vi "PPMS_CREA_SECUENCIA_REPITE.vi"(8 "error in (no error)":errorcluster) -> (0 "error out":errorcluster, 1 "Total":string[](array[string]), 2 "Pasos":i32, 3 "Secuencia":string[](array[string]), 4 "Secuciclos":string[](array[string]), 6 "Pasos f":i32)   [LabVIEW 2017]
uses:
  <vilib>/Utility/file.llb/Read Delimited Spreadsheet (string).vi
panel:
  out "idxScanVi":i16
  out "idxScanVf":i16
  out "Scan V":bool
  out "subArray2D":string[][](array[string])
  out "Seq scans":string[](array[string])
  out "Seq final":string[](array[string])
  out "Seq inicial":string[](array[string])
  out "idxScanTi":i16
  out "idxScanFi":i16
  out "idxScanFf":i16
  out "idxScanTf":i16
  out "Array2D":string[][](array[string])
  out "Scan T":bool
  out "Scan F":bool
  in  "Salir":bool
  in  "Borra linea":bool
  in  "Grabar":bool
  in  "Cargar":bool
  out "SequenceFile":path
  in  "Command line (double click)":i32(listbox) caption="Válvulas"
  in  "Secuencia":i32(listbox)=-1
  # "Noviembre 2020 V1.4  a-sslcdms"
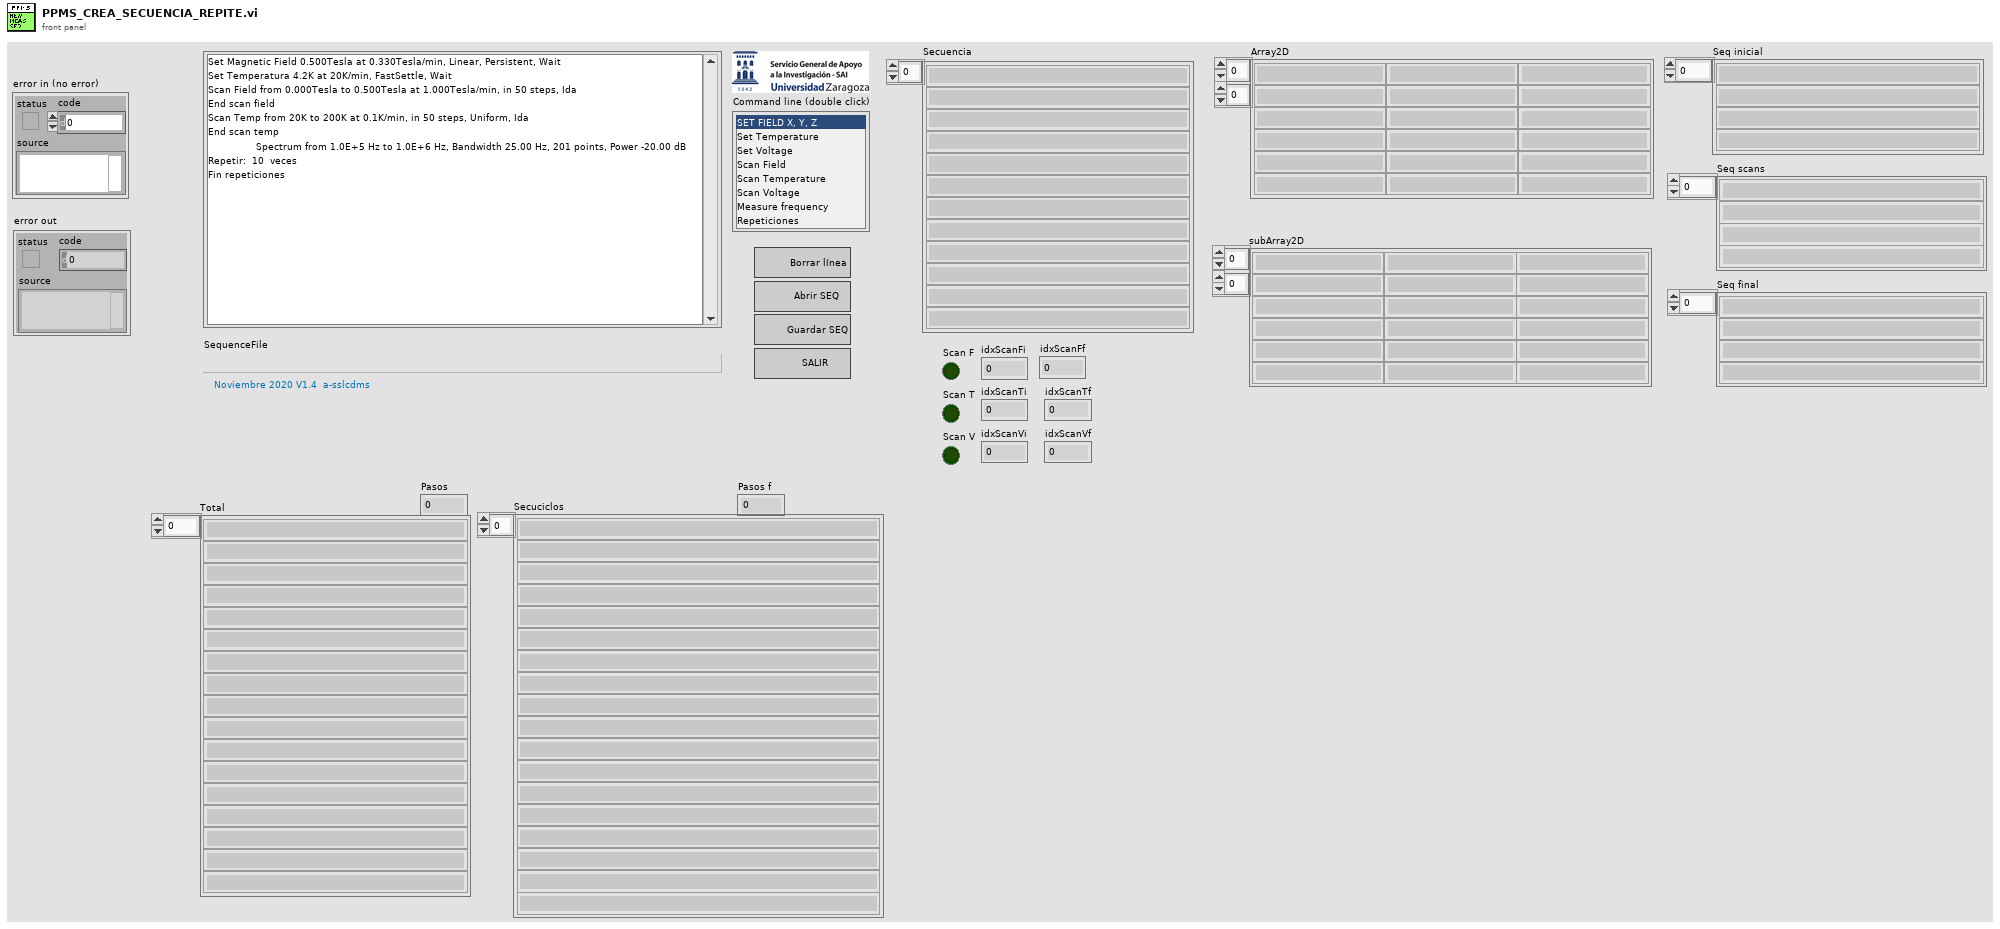
[diagram p1: front panel]
types:
  T1 = enum16{"open", "open or create", "create or replace", "create", "open (read only)"}
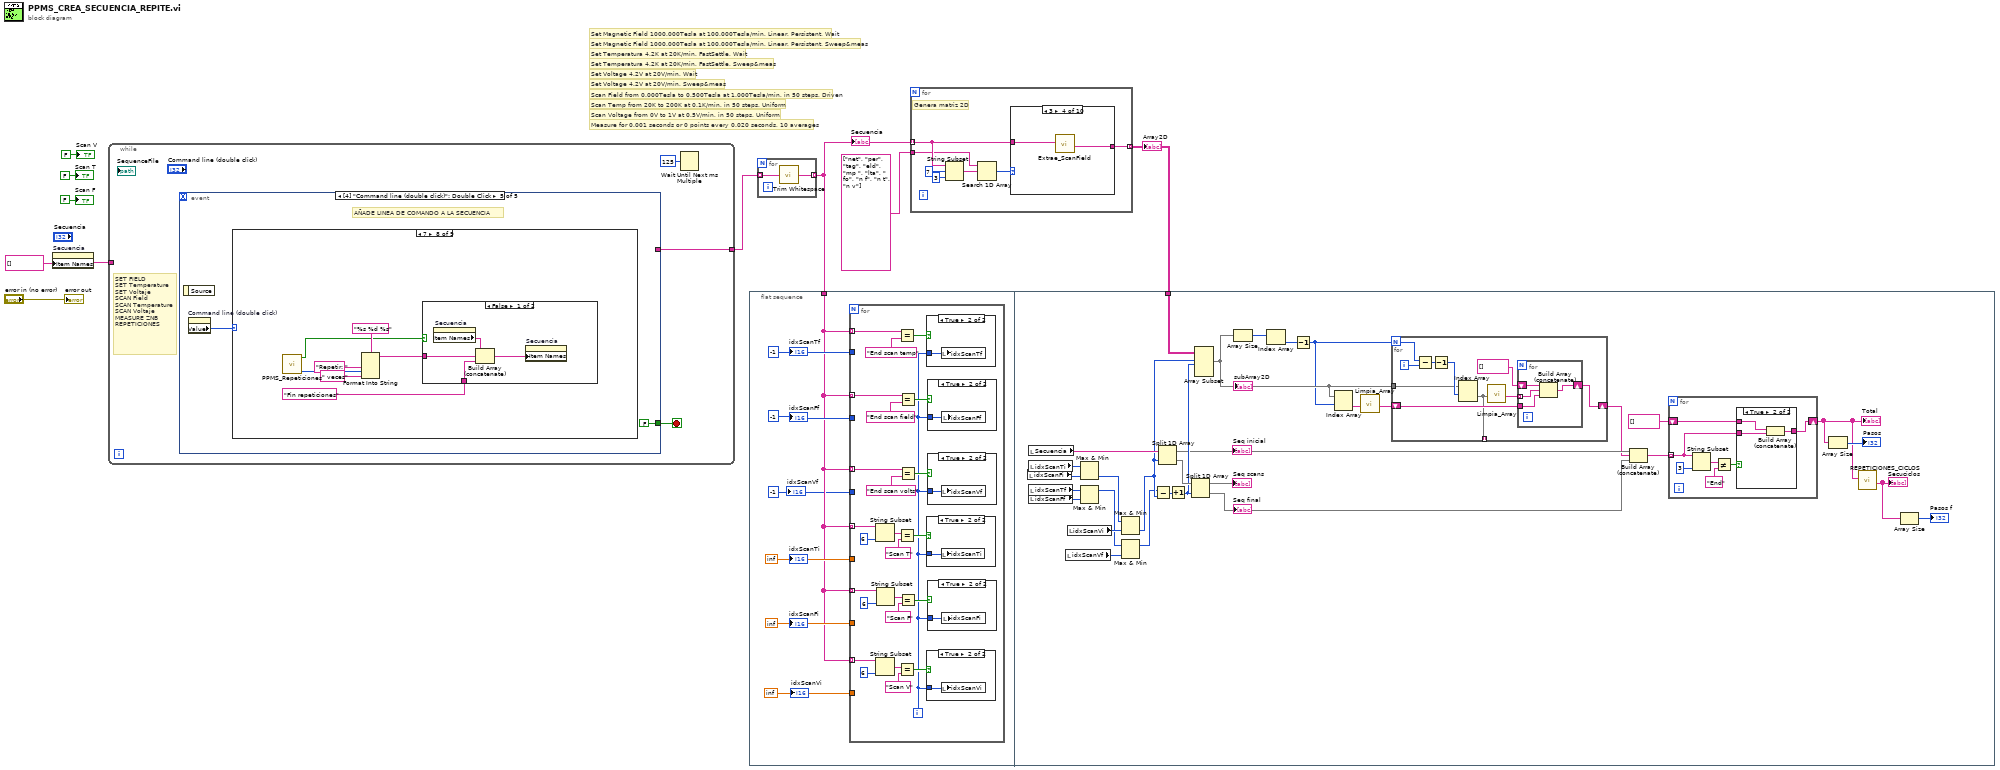
[diagram p0: block diagram]
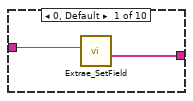
[diagram p9: hidden frame]
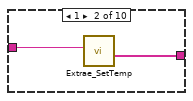
[diagram p10: hidden frame]
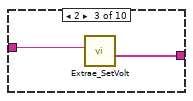
[diagram p11: hidden frame]
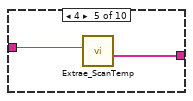
[diagram p12: hidden frame]
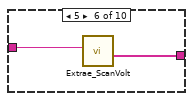
[diagram p13: hidden frame]
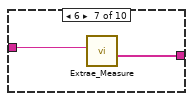
[diagram p14: hidden frame]
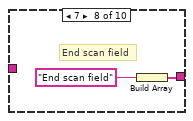
[diagram p15: hidden frame]
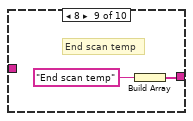
[diagram p16: hidden frame]
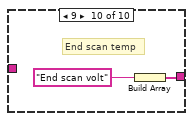
[diagram p17: hidden frame]
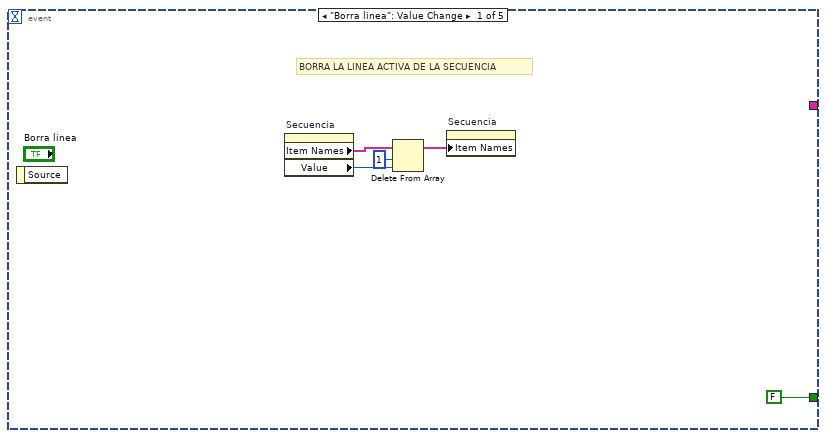
[diagram p18: hidden frame]
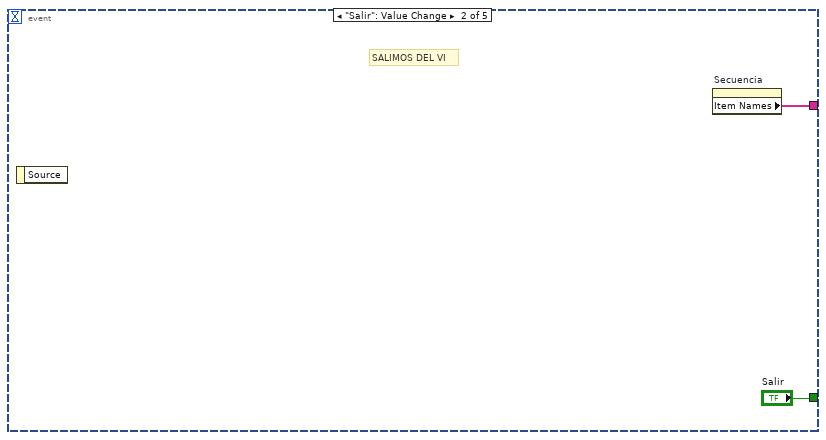
[diagram p19: hidden frame]
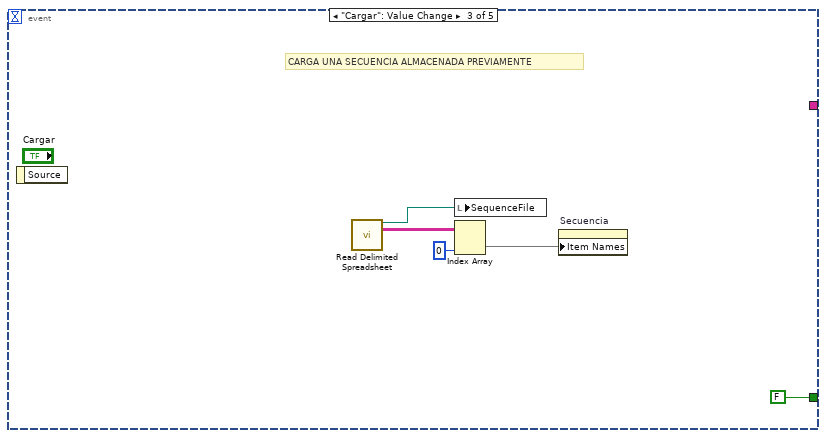
[diagram p20: hidden frame]
diagram:
  w9 = string[] [] ("Item Names")
  # "Measure for 0.001 seconds or 0 points every 0.020 seconds, 10 averages"
  # "Scan Voltage from 0V to 1V at 0.5V/min, in 50 steps, Uniform"
  # "Scan Temp from 20K to 200K at 0.1K/min, in 50 steps, Uniform"
  # "Scan Field from 0.000Tesla to 0.500Tesla at 1.000Tesla/min, in 50 steps, Driven"
  # "Set Temperatura 4.2K at 20K/min, FastSettle, Sweep&meas"
  # "Set Temperatura 4.2K at 20K/min, FastSettle, Wait"
  # "Set Magnetic Field 1000.000Tesla at 100.000Tesla/min, Linear, Persistent, Sweep&meas"
  # "Set Magnetic Field 1000.000Tesla at 100.000Tesla/min, Linear, Persistent, Wait"
  # "Set Voltage 4.2V at 20V/min, Sweep&meas"
  # "Set Voltage 4.2V at 20V/min, Wait"
  n1 = property on="Secuencia" class="LstBox (strict)"("Item Names"=w9) -> ()  [unwired: 2 in, 2 out]
  n2 = while {
    tunnel: w9 -> [_]
    tunnel: [w10] -> w4
    stop <- w11 stop-if-true
    # "SET FIELD\nSET Temperature\nSET Voltaje\nSCAN Field\nSCAN Temperature\nSCAN Voltaje\nMEASURE ZNB\nREPETICIONES"
    n3 = event shown="[4] \"Command line (double click)\": Double Click" {
      selector: _ -> [_ _ _ _ _]
      dyn-events: _ -> [_ _ _ _ _]
      timeout: _ -> [_ _ _ _ _]
      tunnel: [FALSE ("Salir") "Salir" FALSE ("Salir") FALSE ("Salir") FALSE ("Salir")] -> w11
      tunnel: [_ w18 _ _ _] -> w10
      event "Borra linea": Value Change {
        # "BORRA LA LINEA ACTIVA DE LA SECUENCIA"
        n4 = event-data() -> ()  [unwired: 1 in, 1 out]
        n5 = property on="Secuencia" class="LstBox (strict)"() -> ("Item Names"=w17:string[], "Value"=w16:i32)  [unwired: 2 in, 2 out]
        n6 = Delete From Array(array=w17, length=1, index=w16) -> (array with subset deleted=w14:string[])  [unwired: 1 out]
        n7 = property on="Secuencia" class="LstBox (strict)"("Item Names"=w14) -> ()  [unwired: 2 in, 2 out]
      }
      event "Salir": Value Change {
        # "SALIMOS DEL VI"
        n8 = event-data() -> ()  [unwired: 1 in, 1 out]
        n9 = property on="Secuencia" class="LstBox (strict)"() -> ("Item Names"=w18:string[])  [unwired: 2 in, 2 out]
      }
      event "Cargar": Value Change {
        # "CARGA UNA SECUENCIA ALMACENADA PREVIAMENTE"
        n10 = event-data() -> ()  [unwired: 1 in, 1 out]
        n11 = call-poly <vilib>:"Read Delimited Spreadsheet.vi"() -> ("new file path (Not A Path if cancelled)"=w21:path, "all rows"=w20:string[][])  [unwired: 10 in, 4 out]
        n12 = local write "SequenceFile"(w21) -> ()
        n13 = Index Array(array=w20, index (col)=0 ("disabled index (col)")) -> (element=w22:string[])  [unwired: 1 in]
        n14 = property on="Secuencia" class="LstBox (strict)"("Item Names"=w22) -> ()  [unwired: 2 in, 2 out]
      }
      event "Grabar": Value Change {
        # "GRABA UNA SECUENCIA PARA USAR MAS ADELANTE"
        n15 = event-data() -> ()  [unwired: 1 in, 1 out]
        n16 = property on="Secuencia" class="LstBox (strict)"() -> ("Item Names"=w28:string[])  [unwired: 2 in, 2 out]
        n17 = call <vilib>:"Open_Create_Replace File.vi"("function (open:0)"=T1."create or replace") -> ("new file path"=w25:path)  [unwired: 7 in, 3 out]
        n18 = local write "SequenceFile"(w25) -> ()
        n19 = for {
          tunnel: w28 -> [w31] mode=indexing
          shift-right: [w33] -> _
          shift-left: w25 -> [w34]
          n20 = Concatenate Strings(w31, "\r\n") -> (w30:string)
          n21 = call <vilib>:"Write Characters To File.vi"("append to file? (new file:F)"=TRUE, "character string"=w30, "file path (dialog if empty)"=w34) -> ("new file path (Not A Path if cancelled)"=w33:path)  [unwired: 2 in]
        }
      }
      event "Command line (double click)": Double Click {
        # "AÑADE LINEA DE COMANDO A LA SECUENCIA"
        n22 = event-data() -> ()  [unwired: 1 in, 1 out]
        n23 = property on="Command line (double click)" class="LstBox (strict)"() -> ("Value"=w35:i32)  [unwired: 2 in, 2 out]
        n24 = case shown="7" w35 {
          frame 0, Default {
            # "SET FIELD"
            n25 = call "PPMS_SetCampo.vi"("Index"=i8 0) -> ("resulting string 1"=w38:string, "Cancelled?"=w39:bool)  [unwired: 6 in, 1 out]
            n26 = case shown="False" w39 {
              tunnel: w38 -> [w40 _]
              frame False {
                n27 = property on="Secuencia" class="LstBox (strict)"() -> ("Item Names"=w41:string[])  [unwired: 2 in, 2 out]
                n28 = Build Array (concatenate)(w41, w40) -> (w42:string[])
                n29 = property on="Secuencia" class="LstBox (strict)"("Item Names"=w42) -> ()  [unwired: 2 in, 2 out]
              }
              frame True {
              }
            }
          }
          frame 1 {
            # "SET TEMPERATURE"
            n30 = call "PPMS_SetTemperatura.vi"("Index"=i8 0) -> ("resulting string 1"=w44:string, "Cancelled?"=w45:bool)  [unwired: 6 in, 1 out]
            n31 = case shown="False" w45 {
              tunnel: w44 -> [w46 _]
              frame False {
                n32 = property on="Secuencia" class="LstBox (strict)"() -> ("Item Names"=w48:string[])  [unwired: 2 in, 2 out]
                n33 = Build Array (concatenate)(w48, w46) -> (w47:string[])
                n34 = property on="Secuencia" class="LstBox (strict)"("Item Names"=w47) -> ()  [unwired: 2 in, 2 out]
              }
              frame True {
              }
            }
          }
          frame 2 {
            # "SET VOLTAGE"
            n35 = case shown="False" FALSE {
              frame False {
                n36 = One Button Dialog(message="Comando desactivado") -> ()  [unwired: 1 in, 1 out]
              }
              frame True {
                n37 = call "PPMS_SetVoltage.vi"("Index"=i8 0) -> ("resulting string 1"=w51:string, "Cancelled?"=w52:bool)  [unwired: 6 in, 1 out]
                n38 = case shown="False" w52 {
                  tunnel: w51 -> [w56 _]
                  frame False {
                    n39 = property on="Secuencia" class="LstBox (strict)"() -> ("Item Names"=w55:string[])  [unwired: 2 in, 2 out]
                    n40 = Build Array (concatenate)(w55, w56) -> (w54:string[])
                    n41 = property on="Secuencia" class="LstBox (strict)"("Item Names"=w54) -> ()  [unwired: 2 in, 2 out]
                  }
                  frame True {
                  }
                }
              }
            }
          }
          frame 3 {
            # "SCAN FIELD"
            n42 = local read "Scan F"() -> (w57:bool)
            n43 = case shown="False" w57 {
              frame False {
                n44 = local read "Scan T"() -> (w63:bool)
                n45 = local read "Scan V"() -> (w64:bool)
                n46 = Select(t=i8 2 ("Index"), s=w63, f=i8 0 ("Index")) -> (s? t:f=w59:i8)
                n47 = Select(t=i8 2 ("Index"), s=w64, f=i8 0 ("Index")) -> (s? t:f=w60:i8)
                n48 = Add(x=w60, y=w59) -> ()  [unwired: 1 out]
                n49 = local write "Scan F"(TRUE ("Scan T")) -> ()
                n50 = call "PPMS_ScanCampo.vi"("Index"=i8 0) -> ("resulting string 2"=w69:string, "resulting string 1"=w70:string, "Cancelled?"=w68:bool)  [unwired: 5 in, 1 out]
                n51 = case shown="False" w68 {
                  tunnel: w70 -> [w75 _]
                  tunnel: w69 -> [w74 _]
                  frame False {
                    n52 = property on="Secuencia" class="LstBox (strict)"() -> ("Item Names"=w73:string[])  [unwired: 2 in, 2 out]
                    n53 = Build Array(w75, w74) -> (w72:string[])
                    n54 = Build Array (concatenate)(w73, w72) -> (w71:string[])
                    n55 = property on="Secuencia" class="LstBox (strict)"("Item Names"=w71) -> ()  [unwired: 2 in, 2 out]
                  }
                  frame True {
                  }
                }
              }
              frame True {
                n56 = One Button Dialog(message="Solo esta permitido\nun scan de campo por secuencia") -> ()  [unwired: 1 in, 1 out]
              }
            }
          }
          frame 4 {
            # "SCAN TEMPERATURE"
            n57 = local read "Scan T"() -> (w77:bool)
            n58 = case shown="False" w77 {
              frame False {
                n59 = local read "Scan V"() -> (w83:bool)
                n60 = local read "Scan F"() -> (w84:bool)
                n61 = local write "Scan T"(TRUE ("Scan T")) -> ()
                n62 = Select(t=i8 2 ("Index"), s=w83, f=i8 0 ("Index")) -> (s? t:f=w79:i8)
                n63 = Select(t=i8 2 ("Index"), s=w84, f=i8 0 ("Index")) -> (s? t:f=w80:i8)
                n64 = Add(x=w80, y=w79) -> ()  [unwired: 1 out]
                n65 = call "PPMS_ScanTemperatura.vi"("Index"=i8 0) -> ("resulting string 2"=w88:string, "resulting string 1"=w89:string, "Cancelled?"=w90:bool)  [unwired: 5 in, 1 out]
                n66 = case shown="False" w90 {
                  tunnel: w89 -> [w95 _]
                  tunnel: w88 -> [w94 _]
                  frame False {
                    n67 = property on="Secuencia" class="LstBox (strict)"() -> ("Item Names"=w93:string[])  [unwired: 2 in, 2 out]
                    n68 = Build Array(w95, w94) -> (w92:string[])
                    n69 = Build Array (concatenate)(w93, w92) -> (w91:string[])
                    n70 = property on="Secuencia" class="LstBox (strict)"("Item Names"=w91) -> ()  [unwired: 2 in, 2 out]
                  }
                  frame True {
                  }
                }
              }
              frame True {
                n71 = One Button Dialog(message="Solo esta permitido\nun scan de temperatura por secuencia") -> ()  [unwired: 1 in, 1 out]
              }
            }
          }
          frame 5 {
            n72 = case shown="True" FALSE {
              frame False {
                n73 = One Button Dialog(message="Comando desactivado") -> ()  [unwired: 1 in, 1 out]
              }
              frame True {
                # "SCAN VOLTAGE"
                n74 = local read "Scan V"() -> (w99:bool)
                n75 = case shown="False" w99 {
                  frame False {
                    n76 = local read "Scan T"() -> (w107:bool)
                    n77 = local read "Scan F"() -> (w108:bool)
                    n78 = local write "Scan V"(TRUE ("Scan T")) -> ()
                    n79 = Select(t=i8 2 ("Index"), s=w107, f=i8 0 ("Index")) -> (s? t:f=w105:i8)
                    n80 = Select(t=i8 2 ("Index"), s=w108, f=i8 0 ("Index")) -> (s? t:f=w106:i8)
                    n81 = Add(x=w106, y=w105) -> ()  [unwired: 1 out]
                    n82 = call "PPMS_ScanVoltage.vi"("Index"=i8 0) -> ("resulting string 2"=w110:string, "resulting string 1"=w111:string, "Cancelled?"=w112:bool)  [unwired: 5 in, 1 out]
                    n83 = case shown="False" w112 {
                      tunnel: w111 -> [w117 _]
                      tunnel: w110 -> [w116 _]
                      frame False {
                        n84 = property on="Secuencia" class="LstBox (strict)"() -> ("Item Names"=w115:string[])  [unwired: 2 in, 2 out]
                        n85 = Build Array(w117, w116) -> (w114:string[])
                        n86 = Build Array (concatenate)(w115, w114) -> (w113:string[])
                        n87 = property on="Secuencia" class="LstBox (strict)"("Item Names"=w113) -> ()  [unwired: 2 in, 2 out]
                      }
                      frame True {
                      }
                    }
                  }
                  frame True {
                    n88 = One Button Dialog(message="Solo esta permitido\nun scan de temperatura por secuencia") -> ()  [unwired: 1 in, 1 out]
                  }
                }
              }
            }
          }
          frame 6 {
            # "MEASURE CASE  Analizador de frecuencias"
            n89 = local read "Scan V"() -> (w123:bool)
            n90 = local read "Scan T"() -> (w130:bool)
            n91 = local read "Scan F"() -> (w131:bool)
            n92 = Select(t=i8 2 ("Index"), s=w123, f=i8 0 ("Index")) -> (s? t:f=w122:i8)
            n93 = Select(t=i8 2 ("Index"), s=w130, f=i8 0 ("Index")) -> (s? t:f=w126:i8)
            n94 = Select(t=i8 2 ("Index"), s=w131, f=i8 0 ("Index")) -> (s? t:f=w127:i8)
            n95 = Compound Arithmetic op=ADD(w127, w126, w122) -> (w121:i8)
            n96 = call "PPMS_FreqMeas.vi"("Index"=w121) -> ("resulting string 1"=w119:string, "Cancelled?"=w120:bool)  [unwired: 5 in, 2 out]
            n97 = case shown="False" w120 {
              tunnel: w119 -> [w137 _]
              frame False {
                n98 = property on="Secuencia" class="LstBox (strict)"() -> ("Item Names"=w135:string[])  [unwired: 2 in, 2 out]
                n99 = Build Array(w137) -> (w134:string[])
                n100 = Build Array (concatenate)(w135, w134) -> (w136:string[])
                n101 = property on="Secuencia" class="LstBox (strict)"("Item Names"=w136) -> ()  [unwired: 2 in, 2 out]
              }
              frame True {
              }
            }
          }
          frame 7 {
            n102 = call "PPMS_Repeticiones.vi"() -> ("Ciclos"=w139:i32, "Cancelled?"=w138:bool)  [unwired: 10 in]
            n103 = Format Into String(format string="%s %d %s", "Repetir: " ("input 1"), w139, " veces" ("input 3")) -> (resulting string=w144:string)  [unwired: 2 in, 1 out]
            n104 = case shown="False" w138 {
              tunnel: w144 -> [w148 _]
              tunnel: "Fin repeticiones" ("input 1") -> [w147 _]
              frame False {
                n105 = property on="Secuencia" class="LstBox (strict)"() -> ("Item Names"=w146:string[])  [unwired: 2 in, 2 out]
                n106 = Build Array (concatenate)(w146, w148, w147) -> (w145:string[])
                n107 = property on="Secuencia" class="LstBox (strict)"("Item Names"=w145) -> ()  [unwired: 2 in, 2 out]
              }
              frame True {
              }
            }
          }
          frame 8 {
            # "End Program"
            n108 = property on="Secuencia" class="LstBox (strict)"() -> ("Item Names"=w149:string[])  [unwired: 2 in, 2 out]
            n109 = Build Array (concatenate)(w149, "End Program" ("message")) -> ()  [unwired: 1 out]
            n110 = property on="Secuencia" class="LstBox (strict)"("Item Names"=w149) -> ()  [unwired: 2 in, 2 out]
          }
        }
      }
    }
    n111 = Wait Until Next ms Multiple(millisecond multiple=u32 125) -> ()  [unwired: 1 out]
  }
  n112 = flat-sequence {
    tunnel: w3 -> [w153]
    tunnel: w2 -> [w211]
    frame #0 {
      w152 = i16 -1 ("idxScanT")
      w151 = inf
      w154 = inf
      w155 = inf
      w156 = i16 -1 ("idxScanT")
      w157 = i16 -1 ("idxScanT")
      n113 = for {
        tunnel: w153 -> [w173] mode=indexing
        tunnel: w157 -> [_]
        tunnel: w153 -> [w172] mode=indexing
        tunnel: w156 -> [_]
        tunnel: w153 -> [w170] mode=indexing
        tunnel: w153 -> [w169] mode=indexing
        tunnel: w154 -> [_]
        tunnel: w155 -> [_]
        tunnel: w153 -> [w165] mode=indexing
        tunnel: w151 -> [_]
        tunnel: w153 -> [w161] mode=indexing
        tunnel: w152 -> [_]
        i -> [w158]
        n114 = String Subset(string=w170, length (rest)=6 ("length (rest)")) -> (substring=w167:string)  [unwired: 1 in]
        n115 = String Subset(string=w165, length (rest)=6 ("length (rest)")) -> (substring=w166:string)  [unwired: 1 in]
        n116 = String Subset(string=w169, length (rest)=6 ("length (rest)")) -> (substring=w168:string)  [unwired: 1 in]
        n117 = Equal?(x=w173, y="End scan temp" ("trimmed string")) -> (x = y?=w181:bool)
        n118 = Equal?(x=w167, y="Scan T" ("trimmed string")) -> (x = y?=w176:bool)
        n119 = Equal?(x=w166, y="Scan V" ("trimmed string")) -> (x = y?=w163:bool)
        n120 = Equal?(x=w172, y="End scan field" ("trimmed string")) -> (x = y?=w180:bool)
        n121 = Equal?(x=w161, y="End scan volts" ("trimmed string")) -> (x = y?=w159:bool)
        n122 = Equal?(x=w168, y="Scan F" ("trimmed string")) -> (x = y?=w177:bool)
        n123 = case shown="True" w181 {
          tunnel: w158 -> [_ w188]
          frame False {
          }
          frame True {
            n124 = local write "idxScanTf"(w188) -> ()
          }
        }
        n125 = case shown="True" w176 {
          tunnel: w158 -> [_ w186]
          frame False {
          }
          frame True {
            n126 = local write "idxScanTi"(w186) -> ()
          }
        }
        n127 = case shown="True" w163 {
          tunnel: w158 -> [_ w184]
          frame False {
          }
          frame True {
            n128 = local write "idxScanVi"(w184) -> ()
          }
        }
        n129 = case shown="True" w180 {
          tunnel: w158 -> [_ w187]
          frame False {
          }
          frame True {
            n130 = local write "idxScanFf"(w187) -> ()
          }
        }
        n131 = case shown="True" w159 {
          tunnel: w158 -> [_ w183]
          frame False {
          }
          frame True {
            n132 = local write "idxScanVf"(w183) -> ()
          }
        }
        n133 = case shown="True" w177 {
          tunnel: w158 -> [_ w185]
          frame False {
          }
          frame True {
            n134 = local write "idxScanFi"(w185) -> ()
          }
        }
      }
      "idxScanTf" <- w157
      "idxScanFf" <- w156
      "idxScanTi" <- w155
      "idxScanFi" <- w154
      "idxScanVf" <- w152
      "idxScanVi" <- w151
    }
    frame #1 {
      n135 = local read "idxScanFi"() -> (w217:i16)
      n136 = local read "Secuencia"() -> (w219:string[])
      n137 = local read "idxScanTi"() -> (w218:i16)
      n138 = local read "idxScanTf"() -> (w215:i16)
      n139 = local read "idxScanFf"() -> (w216:i16)
      n140 = local read "idxScanVf"() -> (w197:i16)
      n141 = local read "idxScanVi"() -> (w196:i16)
      n142 = Max & Min(x=w218, y=w217) -> (min(x,y)=w195:i16)  [unwired: 1 out]
      n143 = Max & Min(x=w215, y=w216) -> (max(x,y)=w193:i16)  [unwired: 1 out]
      n144 = Max & Min(x=w195, y=w196) -> (min(x,y)=w194:i16)  [unwired: 1 out]
      n145 = Max & Min(x=w193, y=w197) -> (max(x,y)=w192:i16)  [unwired: 1 out]
      n146 = Subtract(x=w192, y=w194) -> (x-y=w212:i16)
      n147 = Split 1D Array(array=w219, index=w194) -> (first subarray=w202:string[], second subarray=w213:string[])
      "Seq inicial" <- w202
      n148 = Increment(x=w212) -> (x+1=w210:i16)
      n149 = Split 1D Array(array=w213, index=w210) -> (first subarray=→"Seq scans":string[], second subarray=w203:string[])
      "Seq final" <- w203
      n150 = Array Subset(array=w211, index (row)=w194, length (row)=w210) -> (w207:string[][])  [unwired: 2 in]
      "subArray2D" <- w207
      n151 = Array Size(array=w207) -> (size(s)=w206:i32[])
      n152 = Index Array(array=w206) -> (element=w205:i32)  [unwired: 1 in]
      n153 = Decrement(x=w205) -> (x-1=w204:i32)
      n154 = Index Array(array=w207, index (row)=w204) -> (element=w208:string[])  [unwired: 1 in]
      n155 = call "Limpia_Array.vi"("Array in"=w208) -> ("Array out"=w209:string[])  [unwired: 10 in]
      n156 = for {
        N: w204 -> [w240]
        tunnel: w207 -> [w237]
        shift-right: [w233] -> w201
        shift-left: w209 -> [w234]
        tunnel: [w231] -> _ mode=indexing
        i -> [w239]
        n157 = Subtract(x=w240, y=w239) -> (x-y=w236:i32)
        n158 = Decrement(x=w236) -> (x-1=w238:i32)
        n159 = Index Array(array=w237, index (row)=w238) -> (element=w231:string[])  [unwired: 1 in]
        n160 = call "Limpia_Array.vi"("Array in"=w231) -> ("Array out"=w232:string[])  [unwired: 10 in]
        n161 = for {
          tunnel: w232 -> [w243] mode=indexing
          shift-right: [w241] -> w233
          shift-left: string[] [] -> [w244]
          tunnel: w234 -> [w242]
          n162 = Build Array (concatenate)(w244, w243, w242) -> (w241:string[])
        }
      }
      n163 = Build Array (concatenate)(w202, w201, w203) -> (w200:string[])
      n164 = for {
        tunnel: w200 -> [w220] mode=indexing
        shift-right: [w222] -> w191
        shift-left: string[] [] -> [w223]
        n165 = String Subset(string=w220, length (rest)=3 ("length (rest)")) -> (substring=w226:string)  [unwired: 1 in]
        n166 = Not Equal?(x=w226, y="End" ("trimmed string")) -> (x != y?=w221:bool)
        n167 = case shown="True" w221 {
          tunnel: w223 -> [w227 w230]
          tunnel: [w227 w229] -> w222
          tunnel: w220 -> [_ w228]
          frame False {
          }
          frame True {
            n168 = Build Array (concatenate)(w230, w228) -> (w229:string[])
          }
        }
      }
      "Total" <- w191
      n169 = Array Size(array=w191) -> (size(s)=→"Pasos":i32)
      n170 = call "REPETICIONES_CICLOS.vi"("Secuencia"=w191) -> ("Secuciclos"=w190:string[])  [unwired: 9 in, 1 out]
      "Secuciclos" <- w190
      n171 = Array Size(array=w190) -> (size(s)=→"Pasos f":i32)
    }
  }
  n172 = for {
    tunnel: w4 -> [w246] mode=indexing
    tunnel: [w245] -> w3 mode=indexing
    n173 = call <vilib>:"Trim Whitespace.vi"("string"=w246) -> ("trimmed string"=w245:string)  [unwired: 1 in]
  }
  "Secuencia" <- w3
  n174 = for {
    tunnel: w3 -> [w248] mode=indexing
    tunnel: [w249] -> w2 mode=indexing
    tunnel: string[] ["net", "per", "tag", "eld", "mp ", "lta", " fo", "n f", "n t", "n v"] ("Array") -> [w247]
    # "Genera matriz 2D"
    n175 = String Subset(string=w248, offset (0)=7, length (rest)=3 ("length (rest)")) -> (substring=w251:string)
    n176 = Search 1D Array(1D array=w247, element=w251) -> (index of element=w250:i32)  [unwired: 1 in]
    n177 = case shown="3" w250 {
      tunnel: w248 -> [w255 w257 w259 w261 w263 w265 w267 _ _ _]
      tunnel: [w254 w256 w258 w260 w262 w264 w266 w268 w270 w272] -> w249
      frame 0, Default {
        n178 = call "Extrae_SetField.vi"("String"=w255) -> ("Array"=w254:string[])  [unwired: 10 in]
      }
      frame 1 {
        n179 = call "Extrae_SetTemp.vi"("String"=w257) -> ("Array"=w256:string[])  [unwired: 10 in]
      }
      frame 2 {
        n180 = call "Extrae_SetVolt.vi"("String"=w259) -> ("Array"=w258:string[])  [unwired: 10 in]
      }
      frame 3 {
        n181 = call "Extrae_ScanField.vi"("F string"=w261) -> ("Array F"=w260:string[])  [unwired: 10 in]
      }
      frame 4 {
        n182 = call "Extrae_ScanTemp.vi"("T string"=w263) -> ("Array T"=w262:string[])  [unwired: 10 in]
      }
      frame 5 {
        n183 = call "Extrae_ScanVolt.vi"("V string"=w265) -> ("Array V"=w264:string[])  [unwired: 10 in]
      }
      frame 6 {
        n184 = call "Extrae_Measure.vi"("String"=w267) -> ("Array"=w266:string[])  [unwired: 10 in]
      }
      frame 7 {
        # "End scan field"
        n185 = Build Array("End scan field" ("trimmed string")) -> (w268:string[])
      }
      frame 8 {
        # "End scan temp"
        n186 = Build Array("End scan temp" ("trimmed string")) -> (w270:string[])
      }
      frame 9 {
        # "End scan temp"
        n187 = Build Array("End scan volt" ("trimmed string")) -> (w272:string[])
      }
    }
  }
  "Array2D" <- w2
  "error out" <- "error in (no error)"
  "Scan F" <- FALSE ("Loop H")
  "Scan T" <- FALSE ("Loop T")
  "Scan V" <- FALSE ("Loop T")
